vi "wa32 GetLastError.vi"(5 "error msg prefix (empty)":string, 7 "generate error (False)":bool, 8 "error in":errorcluster) -> (0 "error out":errorcluster, 2 "error code":u32, 3 "error message":string)   [LabVIEW 2020]
doc: "Retrieves last error code and message from standard WinAPI functions. Can generate error."
uses:
  <vilib>/Utility/error.llb/Error Cluster From Error Code.vi
  <vilib>/ErrorRing/Error Ring.xnode
  kernel32.dll
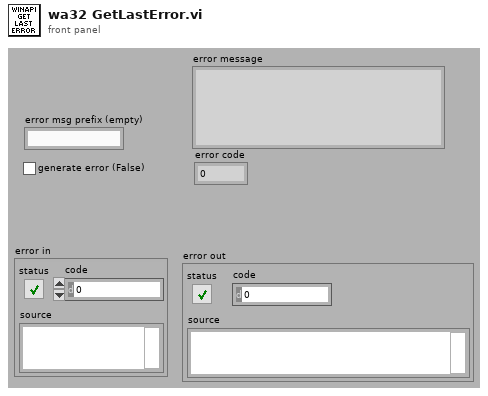
[diagram p1: front panel]
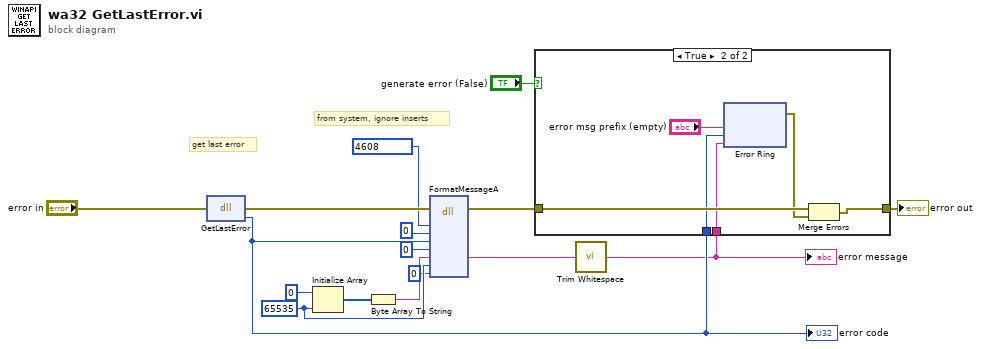
[diagram p0: block diagram]
diagram:
  w9 = 65535 ("dimension size")
  # "get last error"
  # "from system, ignore inserts"
  n1 = dll-call lib="kernel32.dll" fn="GetLastError"(error in="error in") -> (error out=w15:errorcluster, "errout"=w5:u32)  [unwired: 2 in, 1 out]
  "error code" <- w5
  n2 = Initialize Array(u8 0 ("element"), w9) -> (w10:u8[])
  n3 = Byte Array To String(unsigned byte array=w10) -> (string=w2:string)
  n4 = dll-call lib="kernel32.dll" fn="FormatMessageA"(error in=w15, "flags"=u32 4608, "source"=0, "msgID"=w5, "langID"=u32 0, "buffer"=w2, "size"=w9, "vararg"=u32 0 ("arg7")) -> (error out=w8:errorcluster, "buffer"=w1:string)  [unwired: 9 in, 1 out]
  n5 = call <vilib>:"Trim Whitespace.vi"("string"=w1) -> ("trimmed string"=w3:string)  [unwired: 1 in]
  "error message" <- w3
  n6 = case shown="True" "generate error (False)" {
    tunnel: w8 -> [w17 w23]
    tunnel: [w17 w21] -> w7
    tunnel: w3 -> [_ w19]
    tunnel: w5 -> [_ w18]
    frame False {
    }
    frame True {
      n7 = xnode "Error Ring"("parameter 0"="error msg prefix (empty)", "parameter 1"=w18, "parameter 2"=w19) -> ("error out"=w22:errorcluster)
      n8 = Merge Errors(w23, w22) -> (w21:errorcluster)
    }
  }
  "error out" <- w7
